vi "DisableToolbar.vi"(4 "ToolBar.Visible(f)":bool, 6 "FP.ShowMenuBar(f)":bool, 8 "err(in)":errorcluster, 11 "VI入力":refnum<vi>) -> (0 "err(out)":errorcluster, 3 "VI出力":refnum<vi>)   [LabVIEW 2015]
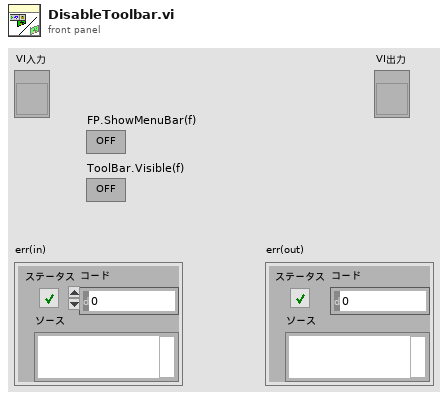
[diagram p1: front panel]
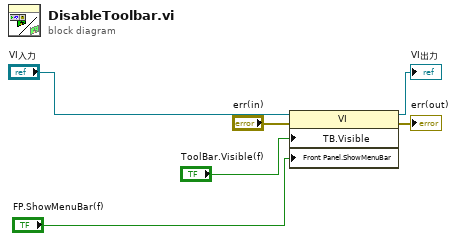
[diagram p0: block diagram]
diagram:
  n1 = property class="VI"(reference="VI入力", error in="err(in)", "TB.Visible"="ToolBar.Visible(f)", "Front Panel.ShowMenuBar"="FP.ShowMenuBar(f)") -> (reference out=→"VI出力":refnum<vi>, error out=→"err(out)":errorcluster)
